vi "valve_actuation.vi"() -> ()   [LabVIEW 2018]
doc: "Manually blink and LED attached to a digital output channel of a LINX device by clicking and LED control in LabVIEW."
uses:
  <vilib>/MakerHub/LINX/Public/Peripherals/Digital/Digital Write 1 Chan.vi
  <vilib>/MakerHub/LINX/Public/Peripherals/Digital/Digital Write N Chans.vi
  <vilib>/MakerHub/LINX/Private/Local IO/LinxDigitalWrite.vi
  <vilib>/MakerHub/LINX/Public/Utilities/Check Channel.vi
  <vilib>/MakerHub/LINX/Public/Utilities/Open Serial.vi
  <vilib>/MakerHub/LINX/Private/Utilties/Generate Error.vi
  <vilib>/MakerHub/LINX/LMH-LINX.lvlib
panel:
  out "id_8":bool
  out "id_7":bool
  out "id_6":bool
  out "id_5":bool
  out "id_4":bool
  out "id_3":bool
  out "id_2":bool
  out "id_1":bool
  in  "stop":bool
  in  "Valve 8":bool
  in  "Valve 7":bool
  in  "Valve 6":bool
  in  "Valve 5":bool
  in  "Valve 4":bool
  in  "Valve 3":bool
  in  "Valve 2":bool
  in  "Valve_1":bool
  in  "Serial Port":refnum<visa-resource-name>
  # "LINX Device Settings"
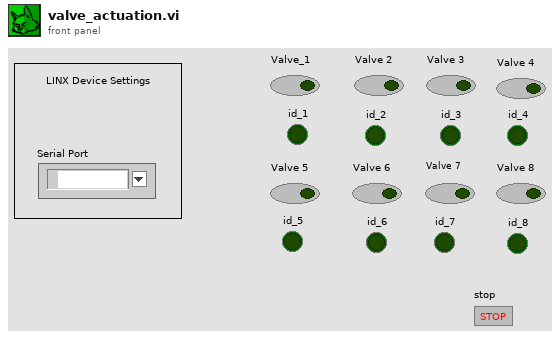
[diagram p1: front panel]
types:
  T1 = typedef "LMH-LINX.lvlib/LINX Ref.ctl" = cluster{"IO":T2, "Interface":T3, "LINX Device Config":T4}
  T2 = typedef "LMH-LINX.lvlib/Platform.ctl" = enum16{"Remote", "Local"}
  T3 = typedef "LMH-LINX.lvlib/Interface.ctl" = enum16{"Serial", "TCP"}
  T4 = typedef "LMH-LINX.lvlib/Device.lvlib/LINX Device Config.ctl" = cluster{"Interface":T3, "COM Port":refnum<visa-resource-name>, "TCP Configuration":T5, "Device Family":u8, "Device ID":u8, "Device Name":string, "TCP Ref":refnum<k5>, "Channels":T6}
  T5 = typedef "LMH-LINX.lvlib/Device.lvlib/TCP Config.ctl" = cluster{"IP Address":string, "Port":u16}
  T6 = typedef "LMH-LINX.lvlib/Channels.ctl" = cluster{"DI":u8[], "DO":u8[], "AI":u8[], "AO":u8[], "PWM":u8[], "QE":u8[], "UART":u8[], "I2C 2":u8[], "SPI":u8[], "CAN":u8[], "Servo":u8[], "AI Ref (V)":dbl, "AI Resolution (Bits)":u8, "AO Ref (V)":dbl, "AO Resolution (Bits)":u8}
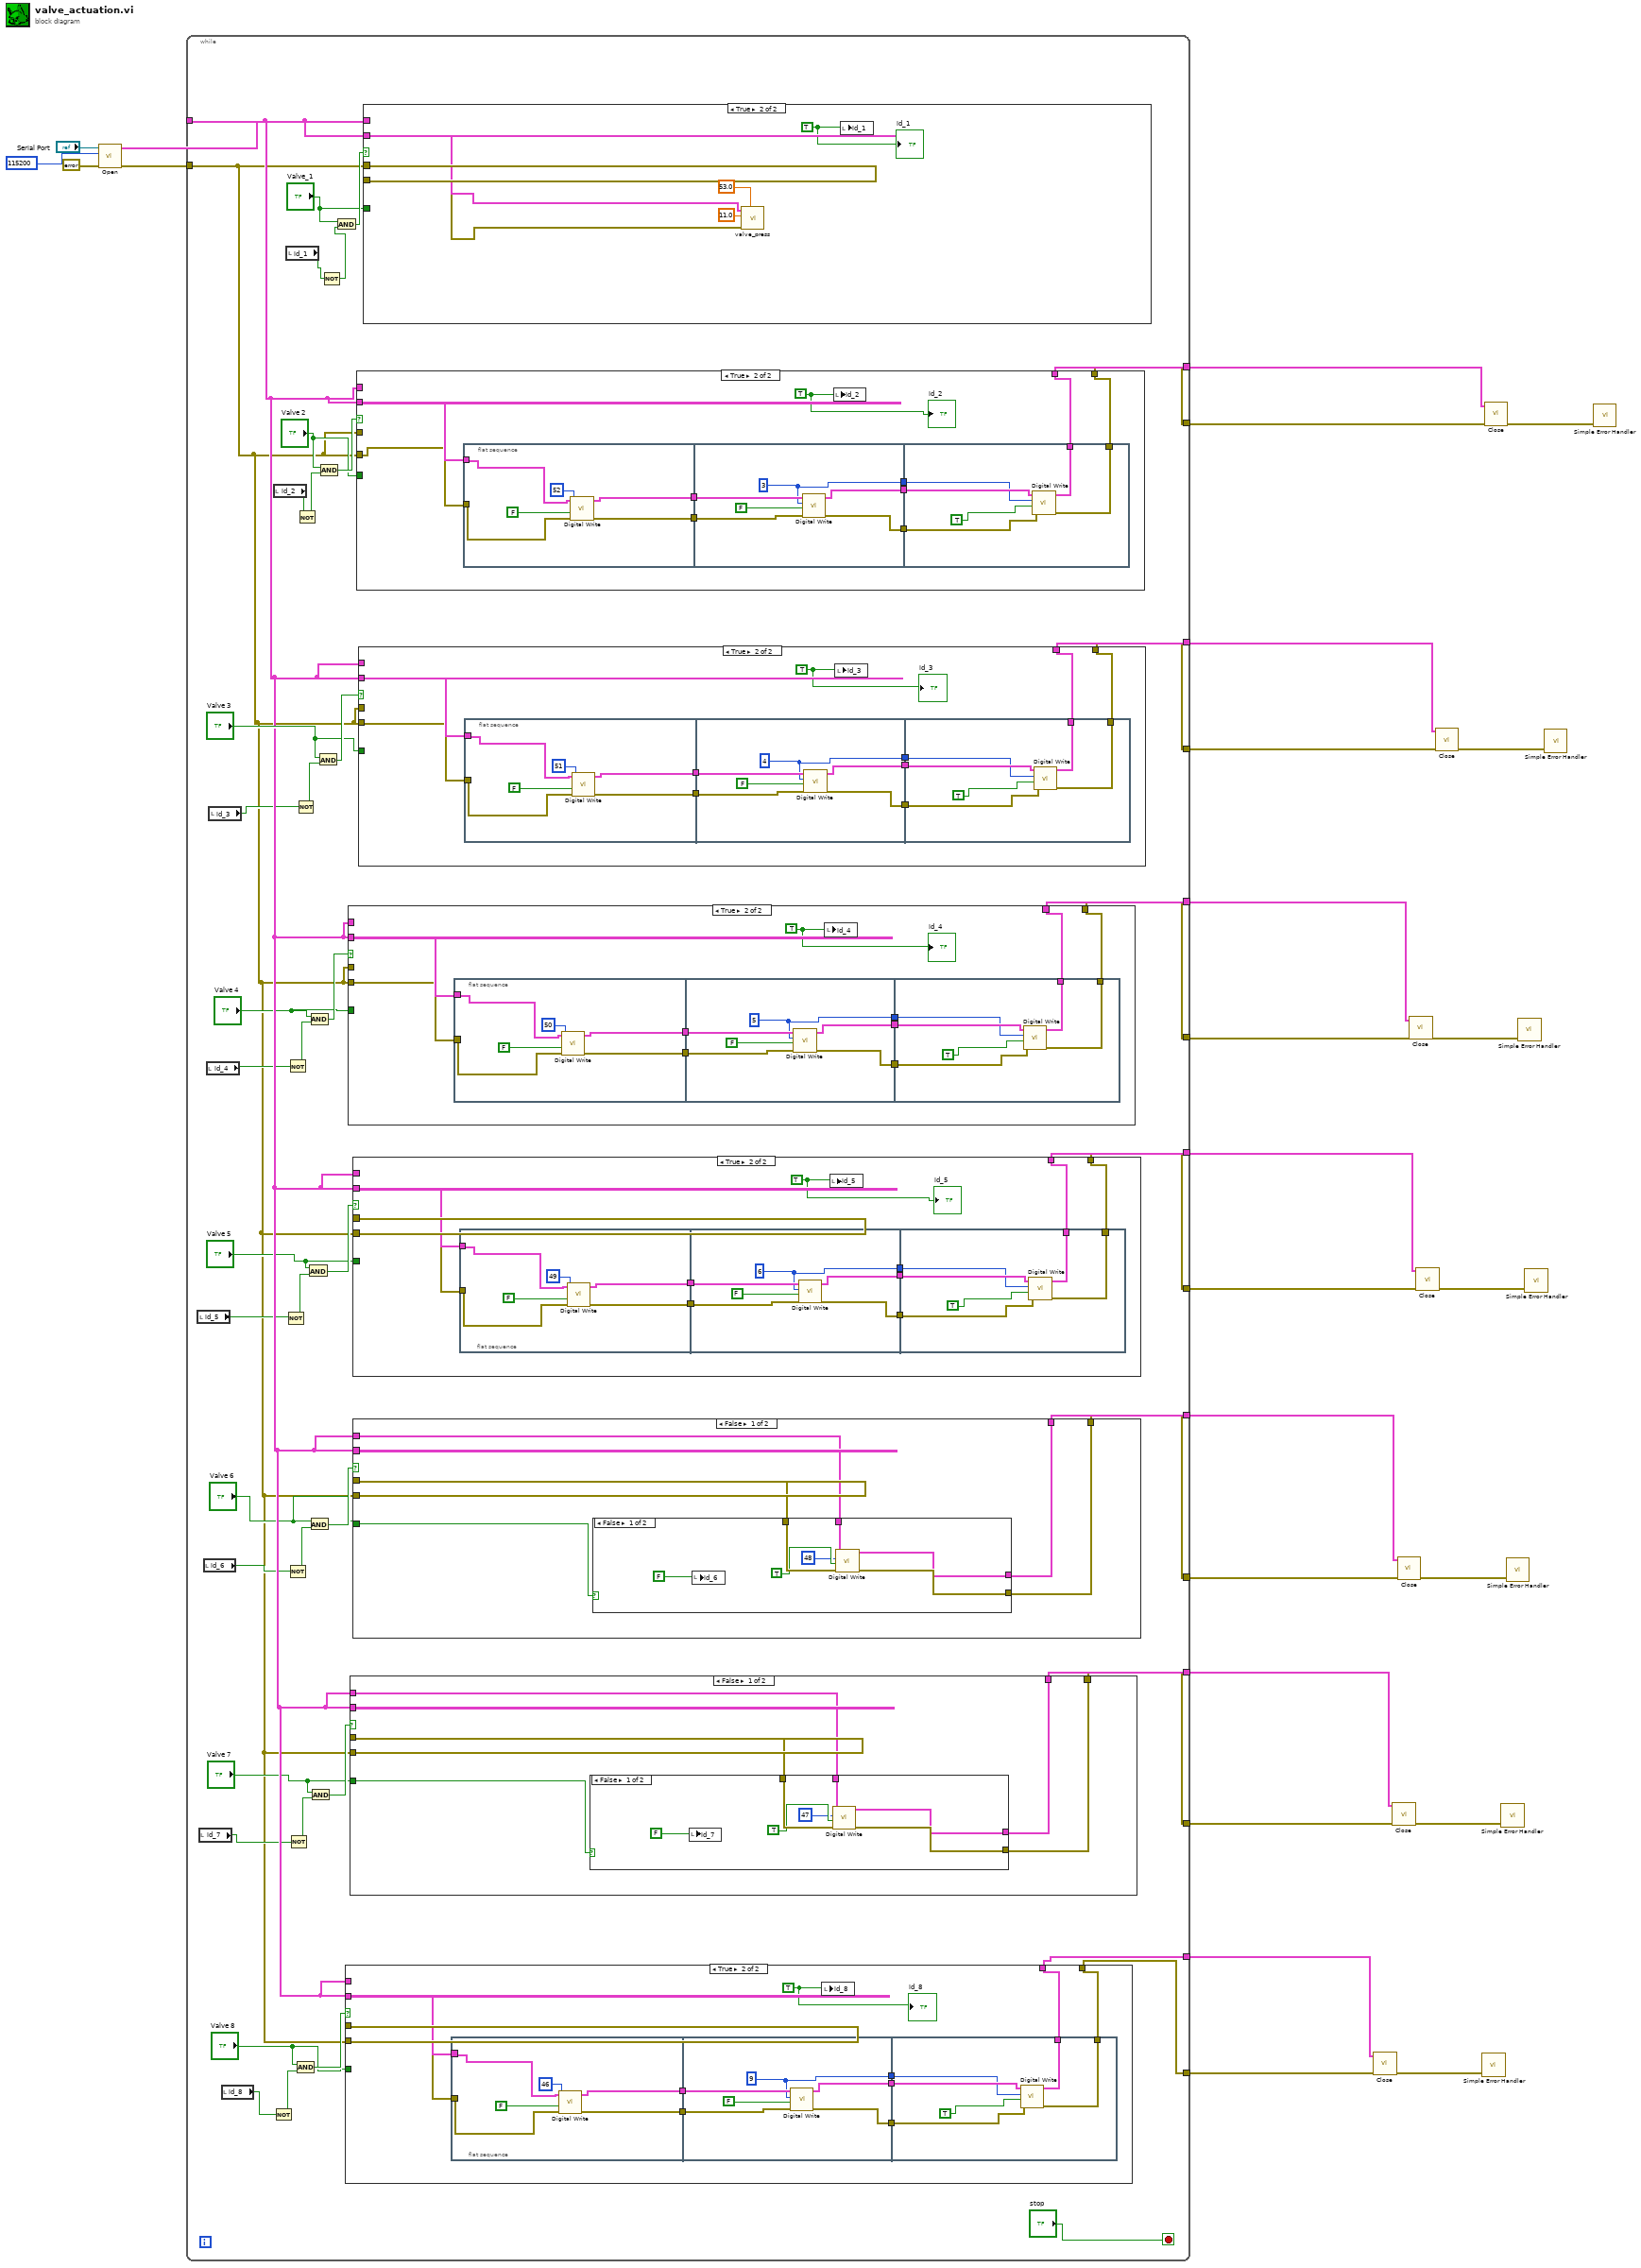
[diagram p0: block diagram]
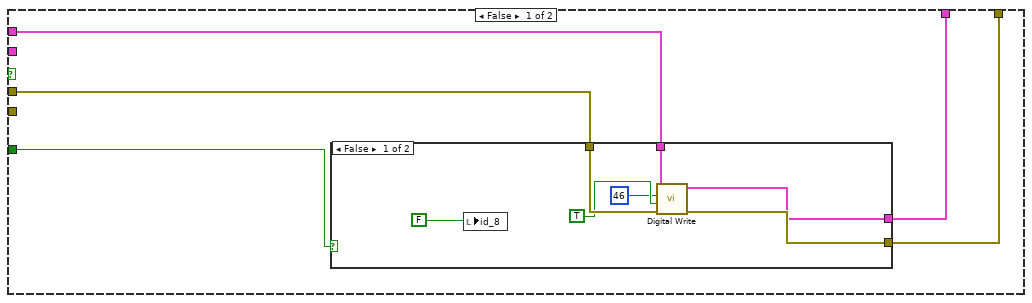
[diagram p2: hidden frame]
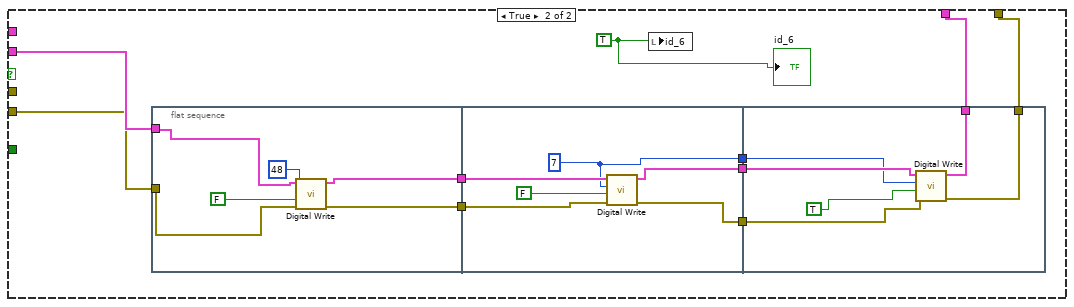
[diagram p5: hidden frame]
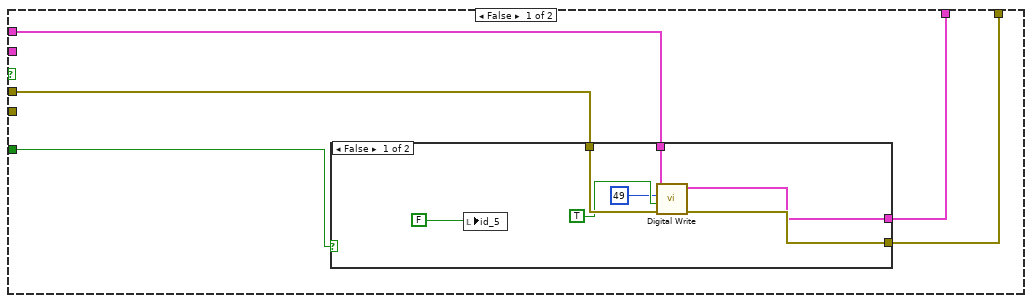
[diagram p6: hidden frame]
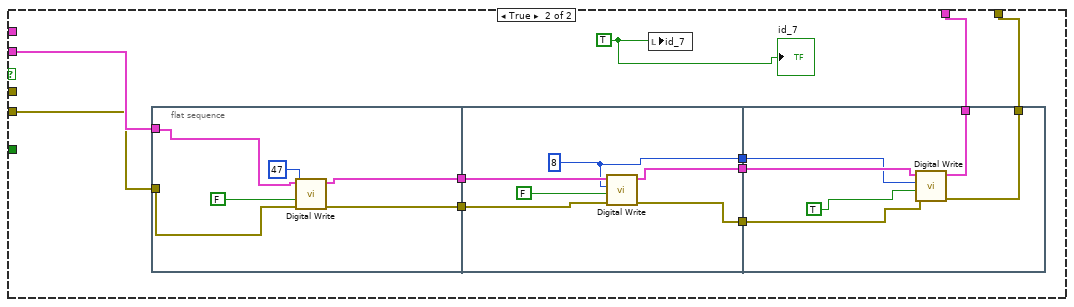
[diagram p9: hidden frame]
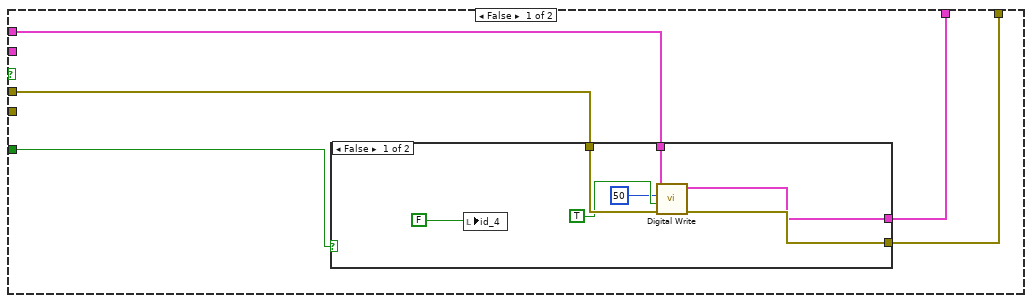
[diagram p10: hidden frame]
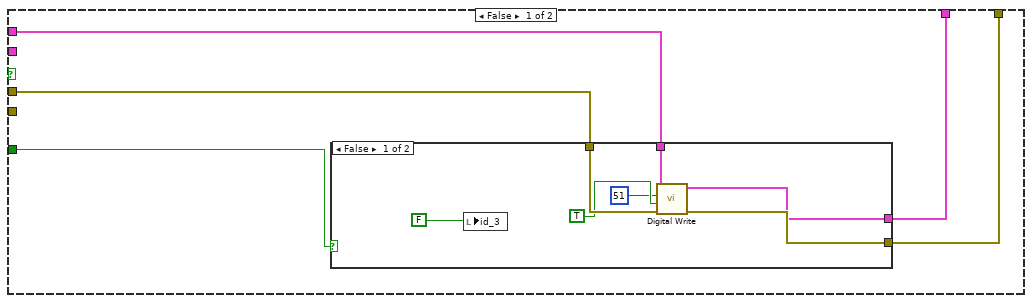
[diagram p12: hidden frame]
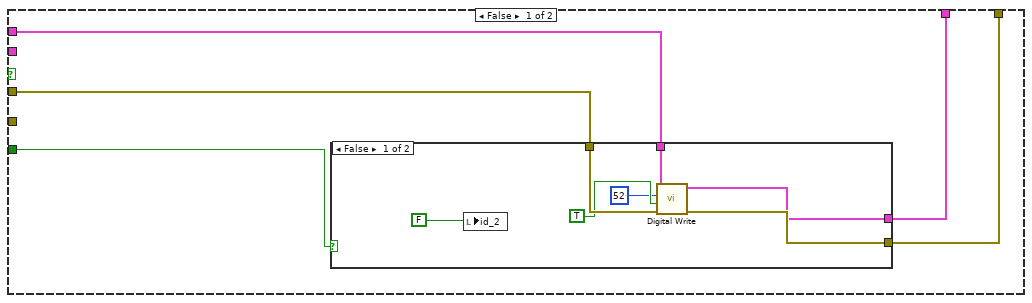
[diagram p14: hidden frame]
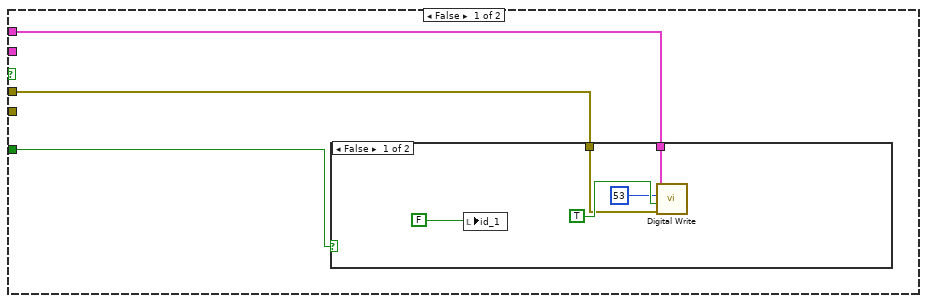
[diagram p16: hidden frame]
diagram:
  n1 = call-poly <vilib>:"Open.vi"("Error In"=errorcluster {"status"=FALSE, "code"=0, "source"=""}, "Baud Rate Override"=u32 115200, "Serial Port"="Serial Port") -> ("Error Out"=w23:errorcluster, "LINX Resource"=w24:T1)  [unwired: 6 in, 1 out]
  n2 = while {
    tunnel: w24 -> [w51]
    tunnel: w23 -> [w27]
    tunnel: [w70] -> w21
    tunnel: [w69] -> w14
    tunnel: [w68] -> w13
    tunnel: [w67] -> w12
    tunnel: [w66] -> w11
    tunnel: [w65] -> w10
    tunnel: [w64] -> w9
    tunnel: [w63] -> w8
    tunnel: [w62] -> w7
    tunnel: [w61] -> w6
    tunnel: [w60] -> w5
    tunnel: [w59] -> w4
    tunnel: [w50] -> w3
    tunnel: [w49] -> w2
    stop <- "stop" stop-if-true
    n3 = local read "id_5"() -> (w44:bool)
    n4 = local read "id_7"() -> (w42:bool)
    n5 = local read "id_6"() -> (w43:bool)
    n6 = local read "id_4"() -> (w45:bool)
    n7 = local read "id_3"() -> (w46:bool)
    n8 = local read "id_8"() -> (w41:bool)
    n9 = Not(x=w41) -> (.not. x?=w40:bool)
    n10 = local read "id_2"() -> (w56:bool)
    n11 = Not(x=w44) -> (.not. x?=w34:bool)
    n12 = local read "id_1"() -> (w73:bool)
    n13 = Not(x=w45) -> (.not. x?=w48:bool)
    n14 = Not(x=w43) -> (.not. x?=w36:bool)
    n15 = Not(x=w42) -> (.not. x?=w38:bool)
    n16 = Not(x=w46) -> (.not. x?=w54:bool)
    n17 = And(x="Valve 8", y=w40) -> (x .and. y?=w39:bool)
    n18 = Not(x=w56) -> (.not. x?=w57:bool)
    n19 = And(x="Valve 5", y=w34) -> (x .and. y?=w33:bool)
    n20 = And(x="Valve 4", y=w48) -> (x .and. y?=w47:bool)
    n21 = And(x="Valve 6", y=w36) -> (x .and. y?=w35:bool)
    n22 = And(x="Valve 7", y=w38) -> (x .and. y?=w37:bool)
    n23 = And(x="Valve 3", y=w54) -> (x .and. y?=w53:bool)
    n24 = And(x="Valve 2", y=w57) -> (x .and. y?=w58:bool)
    n25 = Not(x=w73) -> (.not. x?=w72:bool)
    n26 = And(x="Valve_1", y=w72) -> (x .and. y?=w74:bool)
    n27 = case shown="True" w39 {
      tunnel: w51 -> [_ w99]
      tunnel: w27 -> [_ w98]
      tunnel: [w76 w93] -> w50
      tunnel: [w77 w92] -> w49
      tunnel: "Valve 8" -> [w80 _]
      tunnel: w27 -> [w79 _]
      tunnel: w51 -> [w78 _]
      frame False {
        n28 = case shown="False" w80 {
          tunnel: w79 -> [w86 w88]
          tunnel: w78 -> [w83 w89]
          tunnel: [w82 w88] -> w77
          tunnel: [w81 w89] -> w76
          frame False {
            n29 = local write "id_8"(FALSE) -> ()
            n30 = call-poly <vilib>:"Digital Write.vi"("Error In"=w86, "Output Value"=TRUE, "DO Channel"=u8 46, "LINX Resource"=w83) -> ("Error Out"=w82:errorcluster, "LINX Resource"=w81:T1)  [unwired: 6 in]
          }
          frame True {
          }
        }
      }
      frame True {
        w90 = TRUE
        n31 = flat-sequence {
          tunnel: w99 -> [w100]
          tunnel: w98 -> [w103]
          tunnel: [w102] -> w97
          tunnel: [w101] -> w96
          tunnel: w97 -> [w110]
          tunnel: w96 -> [w109]
          tunnel: [w108] -> w95
          tunnel: [w107] -> w94
          tunnel: [w106] -> w91
          tunnel: w95 -> [w116]
          tunnel: w94 -> [w115]
          tunnel: [w114] -> w93
          tunnel: [w113] -> w92
          tunnel: w91 -> [w112]
          frame #0 {
            n32 = call-poly <vilib>:"Digital Write.vi"("Error In"=w103, "Output Value"=FALSE, "DO Channel"=u8 46, "LINX Resource"=w100) -> ("Error Out"=w101:errorcluster, "LINX Resource"=w102:T1)  [unwired: 6 in]
          }
          frame #1 {
            w106 = u8 9 ("DO Channel")
            n33 = call-poly <vilib>:"Digital Write.vi"("Error In"=w109, "Output Value"=FALSE, "DO Channel"=w106, "LINX Resource"=w110) -> ("Error Out"=w107:errorcluster, "LINX Resource"=w108:T1)  [unwired: 6 in]
          }
          frame #2 {
            n34 = call-poly <vilib>:"Digital Write.vi"("Error In"=w115, "Output Value"=TRUE, "DO Channel"=w112, "LINX Resource"=w116) -> ("Error Out"=w113:errorcluster, "LINX Resource"=w114:T1)  [unwired: 6 in]
          }
        }
        n35 = local write "id_8"(w90) -> ()
        "id_8" <- w90
      }
    }
    n36 = case shown="True" w47 {
      tunnel: w51 -> [_ w267]
      tunnel: w27 -> [_ w266]
      tunnel: [w244 w261] -> w66
      tunnel: [w245 w260] -> w62
      tunnel: "Valve 4" -> [w248 _]
      tunnel: w27 -> [w247 _]
      tunnel: w51 -> [w246 _]
      frame False {
        n37 = case shown="False" w248 {
          tunnel: w247 -> [w254 w256]
          tunnel: w246 -> [w251 w257]
          tunnel: [w250 w256] -> w245
          tunnel: [w249 w257] -> w244
          frame False {
            n38 = local write "id_4"(FALSE) -> ()
            n39 = call-poly <vilib>:"Digital Write.vi"("Error In"=w254, "Output Value"=TRUE, "DO Channel"=u8 50, "LINX Resource"=w251) -> ("Error Out"=w250:errorcluster, "LINX Resource"=w249:T1)  [unwired: 6 in]
          }
          frame True {
          }
        }
      }
      frame True {
        w258 = TRUE
        n40 = flat-sequence {
          tunnel: w267 -> [w268]
          tunnel: w266 -> [w271]
          tunnel: [w270] -> w265
          tunnel: [w269] -> w264
          tunnel: w265 -> [w278]
          tunnel: w264 -> [w277]
          tunnel: [w276] -> w263
          tunnel: [w275] -> w262
          tunnel: [w274] -> w259
          tunnel: w263 -> [w284]
          tunnel: w262 -> [w283]
          tunnel: [w282] -> w261
          tunnel: [w281] -> w260
          tunnel: w259 -> [w280]
          frame #0 {
            n41 = call-poly <vilib>:"Digital Write.vi"("Error In"=w271, "Output Value"=FALSE, "DO Channel"=u8 50, "LINX Resource"=w268) -> ("Error Out"=w269:errorcluster, "LINX Resource"=w270:T1)  [unwired: 6 in]
          }
          frame #1 {
            w274 = u8 5 ("DO Channel")
            n42 = call-poly <vilib>:"Digital Write.vi"("Error In"=w277, "Output Value"=FALSE, "DO Channel"=w274, "LINX Resource"=w278) -> ("Error Out"=w275:errorcluster, "LINX Resource"=w276:T1)  [unwired: 6 in]
          }
          frame #2 {
            n43 = call-poly <vilib>:"Digital Write.vi"("Error In"=w283, "Output Value"=TRUE, "DO Channel"=w280, "LINX Resource"=w284) -> ("Error Out"=w281:errorcluster, "LINX Resource"=w282:T1)  [unwired: 6 in]
          }
        }
        n44 = local write "id_4"(w258) -> ()
        "id_4" <- w258
      }
    }
    n45 = case shown="False" w37 {
      tunnel: w51 -> [_ w225]
      tunnel: w27 -> [_ w224]
      tunnel: [w202 w219] -> w69
      tunnel: [w203 w218] -> w59
      tunnel: "Valve 7" -> [w206 _]
      tunnel: w27 -> [w205 _]
      tunnel: w51 -> [w204 _]
      frame False {
        n46 = case shown="False" w206 {
          tunnel: w205 -> [w212 w214]
          tunnel: w204 -> [w209 w215]
          tunnel: [w208 w214] -> w203
          tunnel: [w207 w215] -> w202
          frame False {
            n47 = local write "id_7"(FALSE) -> ()
            n48 = call-poly <vilib>:"Digital Write.vi"("Error In"=w212, "Output Value"=TRUE, "DO Channel"=u8 47, "LINX Resource"=w209) -> ("Error Out"=w208:errorcluster, "LINX Resource"=w207:T1)  [unwired: 6 in]
          }
          frame True {
          }
        }
      }
      frame True {
        w216 = TRUE
        n49 = flat-sequence {
          tunnel: w225 -> [w226]
          tunnel: w224 -> [w229]
          tunnel: [w228] -> w223
          tunnel: [w227] -> w222
          tunnel: w223 -> [w236]
          tunnel: w222 -> [w235]
          tunnel: [w234] -> w221
          tunnel: [w233] -> w220
          tunnel: [w232] -> w217
          tunnel: w221 -> [w242]
          tunnel: w220 -> [w241]
          tunnel: [w240] -> w219
          tunnel: [w239] -> w218
          tunnel: w217 -> [w238]
          frame #0 {
            n50 = call-poly <vilib>:"Digital Write.vi"("Error In"=w229, "Output Value"=FALSE, "DO Channel"=u8 47, "LINX Resource"=w226) -> ("Error Out"=w227:errorcluster, "LINX Resource"=w228:T1)  [unwired: 6 in]
          }
          frame #1 {
            w232 = u8 8 ("DO Channel")
            n51 = call-poly <vilib>:"Digital Write.vi"("Error In"=w235, "Output Value"=FALSE, "DO Channel"=w232, "LINX Resource"=w236) -> ("Error Out"=w233:errorcluster, "LINX Resource"=w234:T1)  [unwired: 6 in]
          }
          frame #2 {
            n52 = call-poly <vilib>:"Digital Write.vi"("Error In"=w241, "Output Value"=TRUE, "DO Channel"=w238, "LINX Resource"=w242) -> ("Error Out"=w239:errorcluster, "LINX Resource"=w240:T1)  [unwired: 6 in]
          }
        }
        n53 = local write "id_7"(w216) -> ()
        "id_7" <- w216
      }
    }
    n54 = case shown="True" w33 {
      tunnel: w51 -> [_ w183]
      tunnel: w27 -> [_ w182]
      tunnel: [w160 w177] -> w67
      tunnel: [w161 w176] -> w61
      tunnel: "Valve 5" -> [w164 _]
      tunnel: w27 -> [w163 _]
      tunnel: w51 -> [w162 _]
      frame False {
        n55 = case shown="False" w164 {
          tunnel: w163 -> [w170 w172]
          tunnel: w162 -> [w167 w173]
          tunnel: [w166 w172] -> w161
          tunnel: [w165 w173] -> w160
          frame False {
            n56 = local write "id_5"(FALSE) -> ()
            n57 = call-poly <vilib>:"Digital Write.vi"("Error In"=w170, "Output Value"=TRUE, "DO Channel"=u8 49, "LINX Resource"=w167) -> ("Error Out"=w166:errorcluster, "LINX Resource"=w165:T1)  [unwired: 6 in]
          }
          frame True {
          }
        }
      }
      frame True {
        w174 = TRUE
        n58 = flat-sequence {
          tunnel: w183 -> [w184]
          tunnel: w182 -> [w187]
          tunnel: [w186] -> w181
          tunnel: [w185] -> w180
          tunnel: w181 -> [w194]
          tunnel: w180 -> [w193]
          tunnel: [w192] -> w179
          tunnel: [w191] -> w178
          tunnel: [w190] -> w175
          tunnel: w179 -> [w200]
          tunnel: w178 -> [w199]
          tunnel: [w198] -> w177
          tunnel: [w197] -> w176
          tunnel: w175 -> [w196]
          frame #0 {
            n59 = call-poly <vilib>:"Digital Write.vi"("Error In"=w187, "Output Value"=FALSE, "DO Channel"=u8 49, "LINX Resource"=w184) -> ("Error Out"=w185:errorcluster, "LINX Resource"=w186:T1)  [unwired: 6 in]
          }
          frame #1 {
            w190 = u8 6 ("DO Channel")
            n60 = call-poly <vilib>:"Digital Write.vi"("Error In"=w193, "Output Value"=FALSE, "DO Channel"=w190, "LINX Resource"=w194) -> ("Error Out"=w191:errorcluster, "LINX Resource"=w192:T1)  [unwired: 6 in]
          }
          frame #2 {
            n61 = call-poly <vilib>:"Digital Write.vi"("Error In"=w199, "Output Value"=TRUE, "DO Channel"=w196, "LINX Resource"=w200) -> ("Error Out"=w197:errorcluster, "LINX Resource"=w198:T1)  [unwired: 6 in]
          }
        }
        n62 = local write "id_5"(w174) -> ()
        "id_5" <- w174
      }
    }
    n63 = case shown="False" w35 {
      tunnel: w51 -> [_ w141]
      tunnel: w27 -> [_ w140]
      tunnel: [w118 w135] -> w68
      tunnel: [w119 w134] -> w60
      tunnel: "Valve 6" -> [w122 _]
      tunnel: w27 -> [w121 _]
      tunnel: w51 -> [w120 _]
      frame False {
        n64 = case shown="False" w122 {
          tunnel: w121 -> [w128 w130]
          tunnel: w120 -> [w125 w131]
          tunnel: [w124 w130] -> w119
          tunnel: [w123 w131] -> w118
          frame False {
            n65 = local write "id_6"(FALSE) -> ()
            n66 = call-poly <vilib>:"Digital Write.vi"("Error In"=w128, "Output Value"=TRUE, "DO Channel"=u8 48, "LINX Resource"=w125) -> ("Error Out"=w124:errorcluster, "LINX Resource"=w123:T1)  [unwired: 6 in]
          }
          frame True {
          }
        }
      }
      frame True {
        w132 = TRUE
        n67 = flat-sequence {
          tunnel: w141 -> [w142]
          tunnel: w140 -> [w145]
          tunnel: [w144] -> w139
          tunnel: [w143] -> w138
          tunnel: w139 -> [w152]
          tunnel: w138 -> [w151]
          tunnel: [w150] -> w137
          tunnel: [w149] -> w136
          tunnel: [w148] -> w133
          tunnel: w137 -> [w158]
          tunnel: w136 -> [w157]
          tunnel: [w156] -> w135
          tunnel: [w155] -> w134
          tunnel: w133 -> [w154]
          frame #0 {
            n68 = call-poly <vilib>:"Digital Write.vi"("Error In"=w145, "Output Value"=FALSE, "DO Channel"=u8 48, "LINX Resource"=w142) -> ("Error Out"=w143:errorcluster, "LINX Resource"=w144:T1)  [unwired: 6 in]
          }
          frame #1 {
            w148 = u8 7 ("DO Channel")
            n69 = call-poly <vilib>:"Digital Write.vi"("Error In"=w151, "Output Value"=FALSE, "DO Channel"=w148, "LINX Resource"=w152) -> ("Error Out"=w149:errorcluster, "LINX Resource"=w150:T1)  [unwired: 6 in]
          }
          frame #2 {
            n70 = call-poly <vilib>:"Digital Write.vi"("Error In"=w157, "Output Value"=TRUE, "DO Channel"=w154, "LINX Resource"=w158) -> ("Error Out"=w155:errorcluster, "LINX Resource"=w156:T1)  [unwired: 6 in]
          }
        }
        n71 = local write "id_6"(w132) -> ()
        "id_6" <- w132
      }
    }
    n72 = case shown="True" w58 {
      tunnel: w51 -> [_ w351]
      tunnel: [w328 w346] -> w70
      tunnel: [w329 w345] -> w64
      tunnel: "Valve 2" -> [w332 _]
      tunnel: w27 -> [w331 _]
      tunnel: w51 -> [w330 _]
      tunnel: w27 -> [_ w342]
      frame False {
        n73 = case shown="False" w332 {
          tunnel: w331 -> [w338 w340]
          tunnel: w330 -> [w335 w341]
          tunnel: [w334 w340] -> w329
          tunnel: [w333 w341] -> w328
          frame False {
            n74 = local write "id_2"(FALSE) -> ()
            n75 = call-poly <vilib>:"Digital Write.vi"("Error In"=w338, "Output Value"=TRUE, "DO Channel"=u8 52, "LINX Resource"=w335) -> ("Error Out"=w334:errorcluster, "LINX Resource"=w333:T1)  [unwired: 6 in]
          }
          frame True {
          }
        }
      }
      frame True {
        w343 = TRUE
        n76 = flat-sequence {
          tunnel: w351 -> [w352]
          tunnel: w342 -> [w355]
          tunnel: [w354] -> w350
          tunnel: [w353] -> w349
          tunnel: w350 -> [w362]
          tunnel: w349 -> [w361]
          tunnel: [w360] -> w348
          tunnel: [w359] -> w347
          tunnel: [w358] -> w344
          tunnel: w348 -> [w368]
          tunnel: w347 -> [w367]
          tunnel: [w366] -> w346
          tunnel: [w365] -> w345
          tunnel: w344 -> [w364]
          frame #0 {
            n77 = call-poly <vilib>:"Digital Write.vi"("Error In"=w355, "Output Value"=FALSE, "DO Channel"=u8 52, "LINX Resource"=w352) -> ("Error Out"=w353:errorcluster, "LINX Resource"=w354:T1)  [unwired: 6 in]
          }
          frame #1 {
            w358 = u8 3 ("DO Channel")
            n78 = call-poly <vilib>:"Digital Write.vi"("Error In"=w361, "Output Value"=FALSE, "DO Channel"=w358, "LINX Resource"=w362) -> ("Error Out"=w359:errorcluster, "LINX Resource"=w360:T1)  [unwired: 6 in]
          }
          frame #2 {
            n79 = call-poly <vilib>:"Digital Write.vi"("Error In"=w367, "Output Value"=TRUE, "DO Channel"=w364, "LINX Resource"=w368) -> ("Error Out"=w365:errorcluster, "LINX Resource"=w366:T1)  [unwired: 6 in]
          }
        }
        n80 = local write "id_2"(w343) -> ()
        "id_2" <- w343
      }
    }
    n81 = case shown="True" w53 {
      tunnel: w51 -> [_ w309]
      tunnel: w27 -> [_ w308]
      tunnel: [w286 w303] -> w65
      tunnel: [w287 w302] -> w63
      tunnel: "Valve 3" -> [w290 _]
      tunnel: w27 -> [w289 _]
      tunnel: w51 -> [w288 _]
      frame False {
        n82 = case shown="False" w290 {
          tunnel: w289 -> [w296 w298]
          tunnel: w288 -> [w293 w299]
          tunnel: [w292 w298] -> w287
          tunnel: [w291 w299] -> w286
          frame False {
            n83 = local write "id_3"(FALSE) -> ()
            n84 = call-poly <vilib>:"Digital Write.vi"("Error In"=w296, "Output Value"=TRUE, "DO Channel"=u8 51, "LINX Resource"=w293) -> ("Error Out"=w292:errorcluster, "LINX Resource"=w291:T1)  [unwired: 6 in]
          }
          frame True {
          }
        }
      }
      frame True {
        w300 = TRUE
        n85 = flat-sequence {
          tunnel: w309 -> [w310]
          tunnel: w308 -> [w313]
          tunnel: [w312] -> w307
          tunnel: [w311] -> w306
          tunnel: w307 -> [w320]
          tunnel: w306 -> [w319]
          tunnel: [w318] -> w305
          tunnel: [w317] -> w304
          tunnel: [w316] -> w301
          tunnel: w305 -> [w326]
          tunnel: w304 -> [w325]
          tunnel: [w324] -> w303
          tunnel: [w323] -> w302
          tunnel: w301 -> [w322]
          frame #0 {
            n86 = call-poly <vilib>:"Digital Write.vi"("Error In"=w313, "Output Value"=FALSE, "DO Channel"=u8 51, "LINX Resource"=w310) -> ("Error Out"=w311:errorcluster, "LINX Resource"=w312:T1)  [unwired: 6 in]
          }
          frame #1 {
            w316 = u8 4 ("DO Channel")
            n87 = call-poly <vilib>:"Digital Write.vi"("Error In"=w319, "Output Value"=FALSE, "DO Channel"=w316, "LINX Resource"=w320) -> ("Error Out"=w317:errorcluster, "LINX Resource"=w318:T1)  [unwired: 6 in]
          }
          frame #2 {
            n88 = call-poly <vilib>:"Digital Write.vi"("Error In"=w325, "Output Value"=TRUE, "DO Channel"=w322, "LINX Resource"=w326) -> ("Error Out"=w323:errorcluster, "LINX Resource"=w324:T1)  [unwired: 6 in]
          }
        }
        n89 = local write "id_3"(w300) -> ()
        "id_3" <- w300
      }
    }
    n90 = case shown="True" w74 {
      tunnel: w51 -> [_ w379]
      tunnel: w27 -> [_ w378]
      tunnel: "Valve_1" -> [w372 _]
      tunnel: w27 -> [w370 _]
      tunnel: w51 -> [w371 _]
      frame False {
        n91 = case shown="False" w372 {
          tunnel: w371 -> [w374 _]
          tunnel: w370 -> [w373 _]
          frame False {
            n92 = local write "id_1"(FALSE) -> ()
            n93 = call-poly <vilib>:"Digital Write.vi"("Error In"=w373, "Output Value"=TRUE, "DO Channel"=u8 53, "LINX Resource"=w374) -> ()  [unwired: 6 in, 2 out]
          }
          frame True {
          }
        }
      }
      frame True {
        w382 = TRUE
        n94 = call "valve_press.vi"("power"=53.0, "error in (no error)"=w378, "trigger"=11.0, "LINX Resource in"=w379) -> ()  [unwired: 6 in, 2 out]
        n95 = local write "id_1"(w382) -> ()
        "id_1" <- w382
      }
    }
  }
  n96 = call <vilib>:"Close.vi"("Error In"=w2, "LINX Resource"=w3) -> ("Error Out"=w1:errorcluster)  [unwired: 9 in]
  n97 = call <vilib>:"Close.vi"("Error In"=w4, "LINX Resource"=w14) -> ("Error Out"=w15:errorcluster)  [unwired: 9 in]
  n98 = call <vilib>:"Close.vi"("Error In"=w5, "LINX Resource"=w13) -> ("Error Out"=w16:errorcluster)  [unwired: 9 in]
  n99 = call <vilib>:"Close.vi"("Error In"=w7, "LINX Resource"=w11) -> ("Error Out"=w18:errorcluster)  [unwired: 9 in]
  n100 = call <vilib>:"Close.vi"("Error In"=w6, "LINX Resource"=w12) -> ("Error Out"=w17:errorcluster)  [unwired: 9 in]
  n101 = call <vilib>:"Close.vi"("Error In"=w8, "LINX Resource"=w10) -> ("Error Out"=w19:errorcluster)  [unwired: 9 in]
  n102 = call <vilib>:"Simple Error Handler.vi"("error in (no error)"=w1) -> ()  [unwired: 4 in, 5 out]
  n103 = call <vilib>:"Close.vi"("Error In"=w9, "LINX Resource"=w21) -> ("Error Out"=w20:errorcluster)  [unwired: 9 in]
  n104 = call <vilib>:"Simple Error Handler.vi"("error in (no error)"=w15) -> ()  [unwired: 4 in, 5 out]
  n105 = call <vilib>:"Simple Error Handler.vi"("error in (no error)"=w16) -> ()  [unwired: 4 in, 5 out]
  n106 = call <vilib>:"Simple Error Handler.vi"("error in (no error)"=w18) -> ()  [unwired: 4 in, 5 out]
  n107 = call <vilib>:"Simple Error Handler.vi"("error in (no error)"=w17) -> ()  [unwired: 4 in, 5 out]
  n108 = call <vilib>:"Simple Error Handler.vi"("error in (no error)"=w19) -> ()  [unwired: 4 in, 5 out]
  n109 = call <vilib>:"Simple Error Handler.vi"("error in (no error)"=w20) -> ()  [unwired: 4 in, 5 out]
